vi "LogTimestamp.vi"(7 "error in (no error)":errorcluster) -> (0 "error out":errorcluster, 2 "Log Timestamp":string)   [LabVIEW 2017]
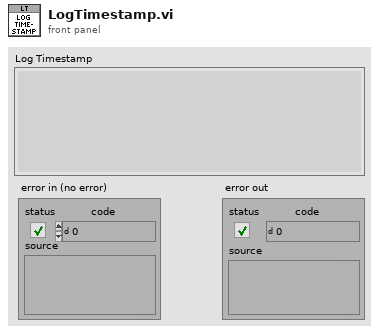
[diagram p1: front panel]
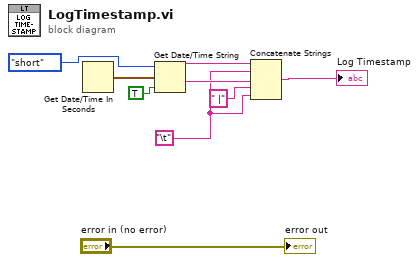
[diagram p0: block diagram]
diagram:
  w1 = "\t"
  n1 = Get Date/Time In Seconds() -> (seconds since 1Jan1904=w5:timestamp)
  n2 = Get Date/Time String(date format (0)=enum16{"short", "long", "abbreviated"}."short", seconds (now)=w5, want seconds? (F)=TRUE) -> (date string=w4:string, time string=w3:string)
  n3 = Concatenate Strings(w4, w1, w3, " |" ("string"), w1) -> (→"Log Timestamp":string)
  "error out" <- "error in (no error)"
